vi "Frequency Dividers.vi"() -> ()   [LabVIEW 2015]
uses:
  <vilib>/gmath/NI_AAL_MathFunc.lvlib
panel:
  out "Found repeats":u32[](array[numeric])=[4, 3, 1, 1]
  out "Posible F":dbl[](array[numeric])=[1190476.1904761905, 1157407.4074074074, 1116071.4285714286, 1041666.6666666666, 992063.4920634921, 925925.925925926, 892857.1428571428, 868055.5555555555, 744047.619047619, 694444.4444444445, 661375.6613756614, 595238.0952380953, 578703.7037037037, 520833.3333333333, 496031.74603174604, 462962.962962963, 446428.5714285714, 396825.3968253968, 372023.8095238095, 347222.22222222225, 330687.8306878307, 297619.04761904763, 289351.85185185185, 248015.87301587302, 231481.4814814815, 223214.2857142857, 198412.6984126984, 173611.11111111112, 165343.91534391535, 148809.52380952382, 132275.1322751323, 124007.93650793651, 115740.74074074074, 99206.3492063492, 82671.95767195767, 74404.76190476191, 66137.56613756614, 57870.37037037037, 49603.1746031746, 41335.978835978836, 33068.78306878307, 24801.5873015873, 16534.391534391536, 8267.195767195768] format="%#_5p"
  out "Bits":u32[](array[numeric])=[7, 7, 7, 7, 7, 8, 8, 8, 8, 8, 8, 8, 8, 8, 8, 9, 9, 9, 9, 9, 9, 9, 9, 9, 10, 10, 10, 10, 10, 10, 10, 10, 11, 11, 11, 11, 11, 12, 12, 12, 12, 13, 13, 14]
  out "Max prime":i64=7
  in  "End factor":i32=16384
  in  "Start factor":i32=100
  in  "Nearest dlock/desired":i64=490
  in  "Max repeat":u32[](array[numeric])=[4, 3, 1, 1]
  out "Points per sine wave":u32[](array[numeric])=[105, 108, 112, 120, 126, 135, 140, 144, 168, 180, 189, 210, 216, 240, 252, 270, 280, 315, 336, 360, 378, 420, 432, 504, 540, 560, 630, 720, 756, 840, 945, 1008, 1080, 1260, 1512, 1680, 1890, 2160, 2520, 3024, 3780, 5040, 7560, 15120]
  out "Prime factors of clock/desired":i64[](array[numeric])=[3, 13, 13]
  out "Clock/Desired":dbl=482.6254826254826
  in  "Desired frequency":dbl=259000.0 format="%#_8p"
  in  "Clock frequency":dbl=125000000.0 format="%#_8p"
  out "Max product log2+1 (bit size)":u32=14
  out "Phase acumulator modulus":i64=15120 format="%d (0x%x)"
  in  "Factors":i64[](array[numeric])=[2, 3, 5, 7]
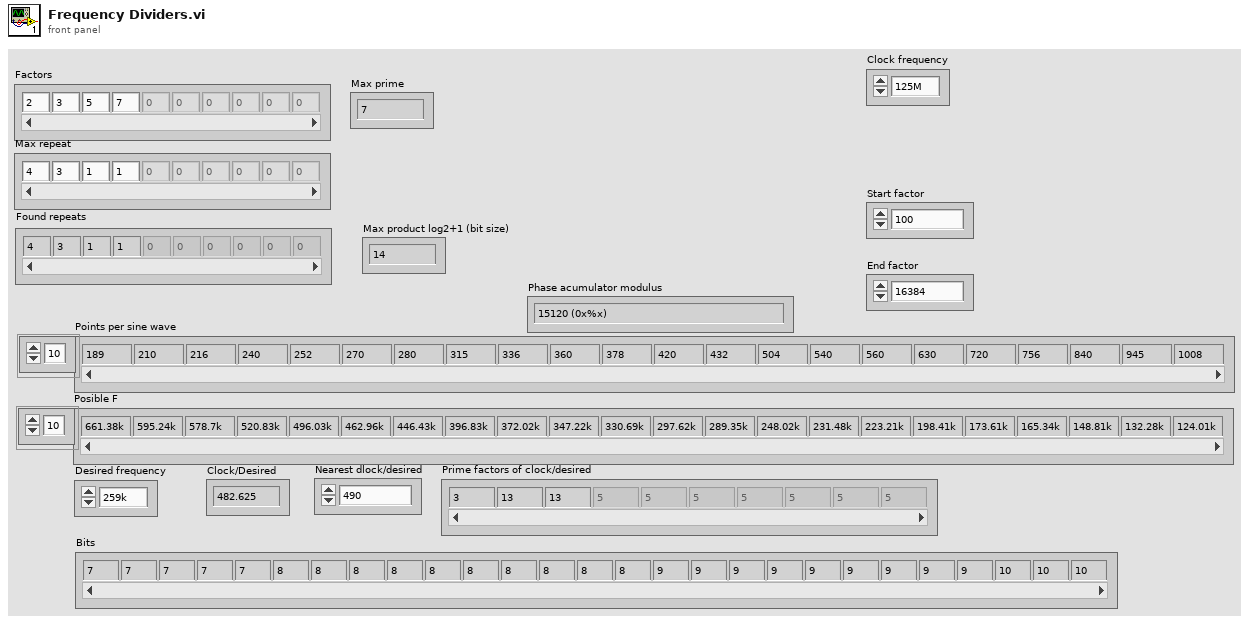
[diagram p1: front panel]
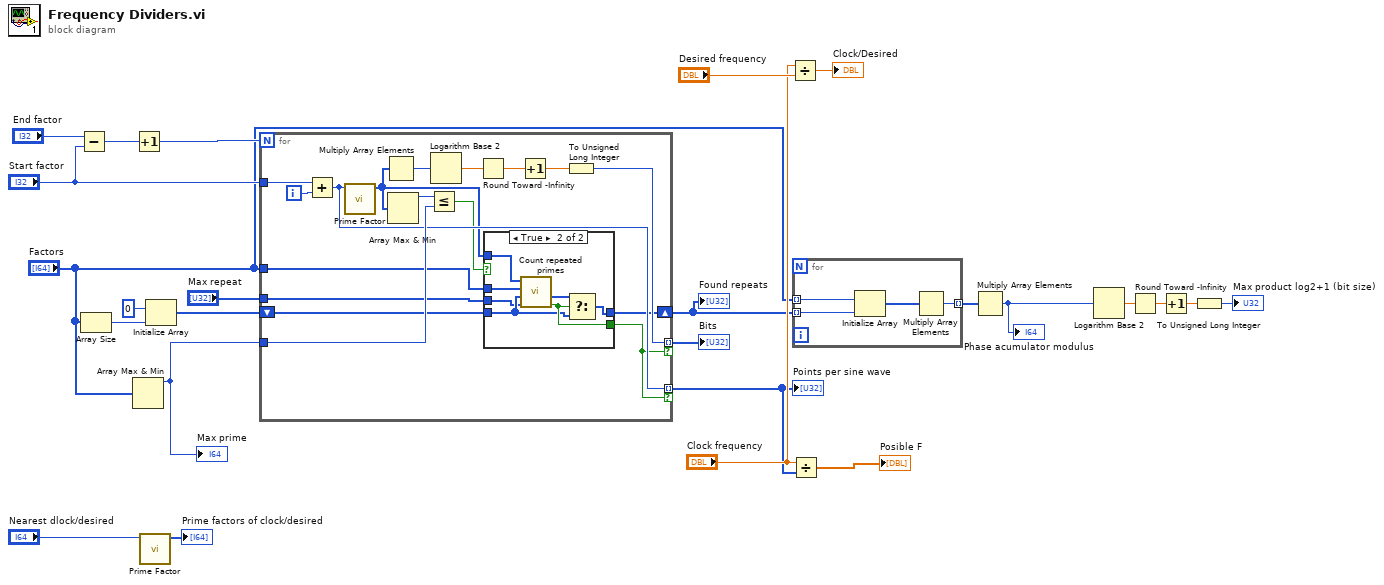
[diagram p0: block diagram]
diagram:
  n1 = Subtract(x="End factor", y="Start factor") -> (x-y=w14:i32)
  n2 = Array Size(array="Factors") -> (size(s)=w7:i32)
  n3 = Array Max & Min(array="Factors") -> (max value=w1:i64)  [unwired: 3 out]
  "Max prime" <- w1
  n4 = Increment(x=w14) -> (x+1=w13:i32)
  n5 = call <vilib>:"Prime Factor.vi"("n"="Nearest dlock/desired") -> ("Prime Factors"=→"Prime factors of clock/desired":i64[])  [unwired: 9 in]
  n6 = Initialize Array(0, w7) -> (w5:i32[])
  n7 = for {
    N: w13 -> [_]
    tunnel: "Start factor" -> [w42]
    tunnel: w1 -> [w40]
    tunnel: [w38] -> w9 mode=indexing if=w27
    tunnel: [w33] -> w11 mode=indexing if=w27
    tunnel: "Factors" -> [w31]
    shift-right: [w29] -> w3
    shift-left: w5 -> [w30]
    tunnel: "Max repeat" -> [w26]
    i -> [w39]
    n8 = Add(x=w42, y=w39) -> (x+y=w38:i32)
    n9 = call <vilib>:"Prime Factor.vi"("n"=w38) -> ("Prime Factors"=w32:i64[])  [unwired: 9 in]
    n10 = Multiply Array Elements(1:w32) -> (0:w34:i64)
    n11 = Array Max & Min(array=w32) -> (max value=w41:i64)  [unwired: 3 out]
    n12 = Less Or Equal?(x=w41, y=w40) -> (x <= y?=w28:bool)
    n13 = Logarithm Base 2(1:w34) -> (0:w35:dbl)
    n14 = Round Toward -Infinity(1:w35) -> (0:w36:dbl)
    n15 = case shown="True" w28 {
      selector: w28 -> [w43 _]
      tunnel: w32 -> [_ w51]
      tunnel: w31 -> [_ w50]
      tunnel: w30 -> [w44 w47]
      tunnel: [w44 w46] -> w29
      tunnel: [w43 w49] -> w27
      tunnel: w26 -> [_ w45]
      frame False {
      }
      frame True {
        n16 = call "Count repeated primes.vi"("Max total"=w45, "Previous total"=w47, "Numbers to look for"=w50, "Array"=w51) -> ("Below max reps"=w49:bool, "Total found"=w48:i32[])  [unwired: 5 in, 1 out]
        n17 = Select(t=w48, s=w49, f=w47) -> (s? t:f=w46:i32[])
      }
    }
    n18 = Increment(x=w36) -> (x+1=w37:dbl)
    n19 = To Unsigned Long Integer(number=w37) -> (unsigned 32bit integer=w33:u32)
  }
  "Points per sine wave" <- w9
  "Bits" <- w11
  "Found repeats" <- w3
  n20 = Divide(x="Clock frequency", y="Desired frequency") -> (x/y=→"Clock/Desired":dbl)
  n21 = Divide(x="Clock frequency", y=w9) -> (x/y=→"Posible F":dbl[])
  n22 = for {
    tunnel: w3 -> [w54] mode=indexing
    tunnel: "Factors" -> [w55] mode=indexing
    tunnel: [w52] -> w17 mode=indexing
    n23 = Initialize Array(w55, w54) -> (w53:i64[])
    n24 = Multiply Array Elements(1:w53) -> (0:w52:i64)
  }
  n25 = Multiply Array Elements(1:w17) -> (0:w25:i64)
  "Phase acumulator modulus" <- w25
  n26 = Logarithm Base 2(1:w25) -> (0:w24:dbl)
  n27 = Round Toward -Infinity(1:w24) -> (0:w23:dbl)
  n28 = Increment(x=w23) -> (x+1=w22:dbl)
  n29 = To Unsigned Long Integer(number=w22) -> (unsigned 32bit integer=→"Max product log2+1 (bit size)":u32)
